vi "onNewHttpSession.vi"(6 "verify server (true)":bool, 7 "cookie file":path, 8 "error in (no error)":errorcluster, 9 "password":string, 10 "username":string, 11 "REST Client in":refnum<class "REST Client.lvclass">) -> (0 "error out":errorcluster, 3 "REST Client out":refnum<class "REST Client.lvclass">)   [LabVIEW 2020, in "REST Client.lvlib" / "REST Client.lvclass"]
uses:
  REST Client.lvclass
  REST Client.lvclass/REST Client.ctl
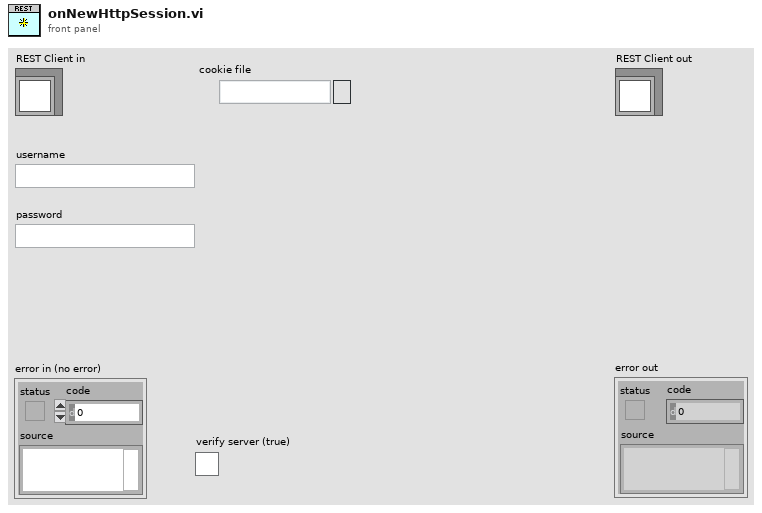
[diagram p1: front panel]
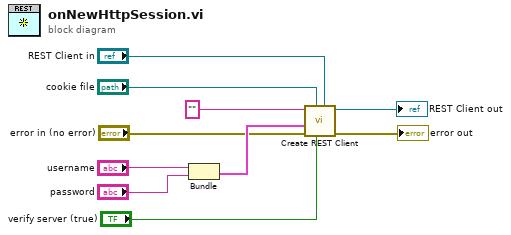
[diagram p0: block diagram]
diagram:
  n1 = Bundle("username"="username", "password"="password") -> (w4:cluster{"username":string, "password":string})  [unwired: 1 in]
  n2 = call "Create REST Client.vi"("REST Client in"="REST Client in", "Verify Server(true)"="verify server (true)", "Cookie File"="cookie file", "error in (no error)"="error in (no error)", "Authentication"=w4, "Base URL"="") -> ("error out"=→"error out":errorcluster, "REST Client out"=→"REST Client out":refnum<class "REST Client.lvclass">)  [unwired: 4 in]
